vi "holoTrackPath.vi"() -> (3 "appended path":path)   [LabVIEW 2025, in "holoTracker.lvlib"]
uses:
  holoTracker.lvlib
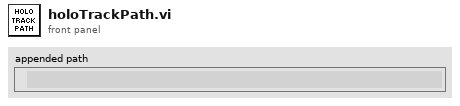
[diagram p1: front panel]
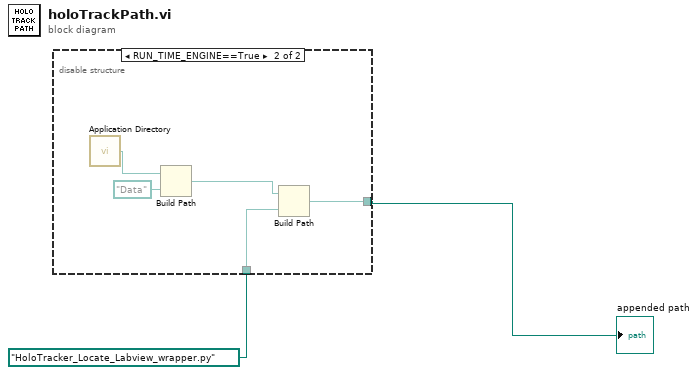
[diagram p0: block diagram]
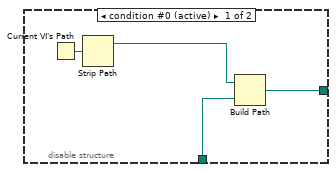
[diagram p2: hidden frame]
diagram:
  n1 = disable-structure shown="RUN_TIME_ENGINE==True" {
    disable-tunnel: [w4 w11] -> w2
    disable-tunnel: path "HoloTracker_Locate_Labview_wrapper.py" ("name or relative path") -> [w3 w10]
    frame condition #0 (active) {
      n2 = Current VI's Path() -> (path=w5:path)
      n3 = Strip Path(path=w5) -> (stripped path=w6:path)  [unwired: 1 out]
      n4 = Build Path(base path=w6, name or relative path=w3) -> (appended path=w4:path)
    }
    frame condition #1 {
      n5 = call <vilib>:"Application Directory.vi"() -> ("Application Directory"=w9:path)
      n6 = Build Path(base path=w9, name or relative path=path "Data") -> (appended path=w7:path)
      n7 = Build Path(base path=w7, name or relative path=w10) -> (appended path=w11:path)
    }
  }
  "appended path" <- w2
